vi "Fwd Kenimatics - array.vi"(4 "To":i32=7, 7 "From":i32=-1, 8 "Side":T1=enum."right", 11 "Joints":dbl[](array[numeric])=[0.0, 0.0, 0.0, 0.0, 0.0, -0.0, 0.0]) -> (0 "Matrix":T2 format="%.3f", 3 "Position":dbl[](array[numeric]) format="%.3f")   [LabVIEW 2013]
uses:
  <vilib>/Analysis/Matrix/Datatypes/RealMatrix.ctl
  ROS/Code/SubVIs/BaxterSide.ctl
  <vilib>/Analysis/Matrix/Numeric/Conversions/Array To Matrix - RA2.vi
  <vilib>/Analysis/Matrix/Numeric/Conversions/Matrix To Array - RM.vi
  <vilib>/Analysis/Matrix/Numeric/Multiply/Multiply - RM,RM.vi
  <vilib>/Analysis/Matrix/NI_Matrix.lvlib
panel:
  out "Individual":dbl[][][](array[numeric])=[[[1.0, 0.0, 0.0, 69.0], [0.0, 6.123233995736766e-17, 1.0, 0.0], [0.0, -1.0, 6.123233995736766e-17, 270.35], [0.0, 0.0, 0.0, 1.0]], [[6.123233995736766e-17, -6.123233995736766e-17, 1.0, 0.0], [1.0, 3.749399456654644e-33, -6.123233995736766e-17, 0.0], [0.0, 1.0, 6.123233995736766e-17, 0.0], [0.0, 0.0, 0.0, 1.0]], [[1.0, 0.0, 0.0, 69.0], [0.0, 6.123233995736766e-17, 1.0, 0.0], [0.0, -1.0, 6.123233995736766e-17, 364.35], [0.0, 0.0, 0.0, 1.0]], [[1.0, 0.0, 0.0, 0.0], [0.0, 6.123233995736766e-17, -1.0, 0.0], [0.0, 1.0, 6.123233995736766e-17, 0.0], [0.0, 0.0, 0.0, 1.0]], [[1.0, 0.0, 0.0, 10.0], [0.0, 6.123233995736766e-17, 1.0, 0.0], [0.0, -1.0, 6.123233995736766e-17, 374.29], [0.0, 0.0, 0.0, 1.0]], [[1.0, 0.0, 0.0, 0.0], [0.0, 6.123233995736766e-17, -1.0, 0.0], [0.0, 1.0, 6.123233995736766e-17, 0.0], [0.0, 0.0, 0.0, 1.0]], [[1.0, 0.0, 0.0, 0.0], [0.0, 1.0, 0.0, 0.0], [0.0, 0.0, 1.0, 229.525], [0.0, 0.0, 0.0, 1.0]]] format="%.3f"
  in  "D-H":cluster{"D":dbl, "R":dbl, "Rz":dbl, "Rx":dbl}[](array[cluster])=[{"D"=270.35, "R"=69.0, "Rz"=0.0, "Rx"=-90.0}, {"D"=0.0, "R"=0.0, "Rz"=90.0, "Rx"=90.0}, {"D"=364.35, "R"=69.0, "Rz"=0.0, "Rx"=-90.0}, {"D"=0.0, "R"=0.0, "Rz"=0.0, "Rx"=90.0}, {"D"=374.29, "R"=10.0, "Rz"=0.0, "Rx"=-90.0}, {"D"=0.0, "R"=0.0, "Rz"=0.0, "Rx"=90.0}, {"D"=229.525, "R"=0.0, "Rz"=0.0, "Rx"=0.0}]
  # "Does not include gripper\nFrom Base to Tool Plate"
  # "0->1\n\n1->2\n\n2->3\n\n3->4\n\n4->5\n\n5->6\n\n6->gripper"
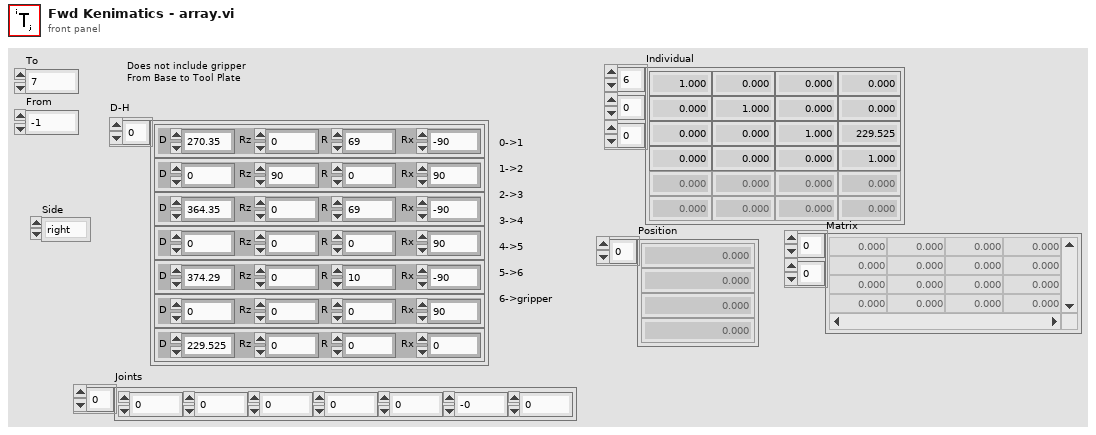
[diagram p1: front panel]
types:
  T1 = typedef "BaxterSide.ctl" = enum16{"left", "right"}
  T2 = typedef "NI_Matrix.lvlib/RealMatrix.ctl" = dbl[][]
  T3 = cluster{"Real Matrix":T2, "Real Matrix":T2, "A * B":dbl[][][]}
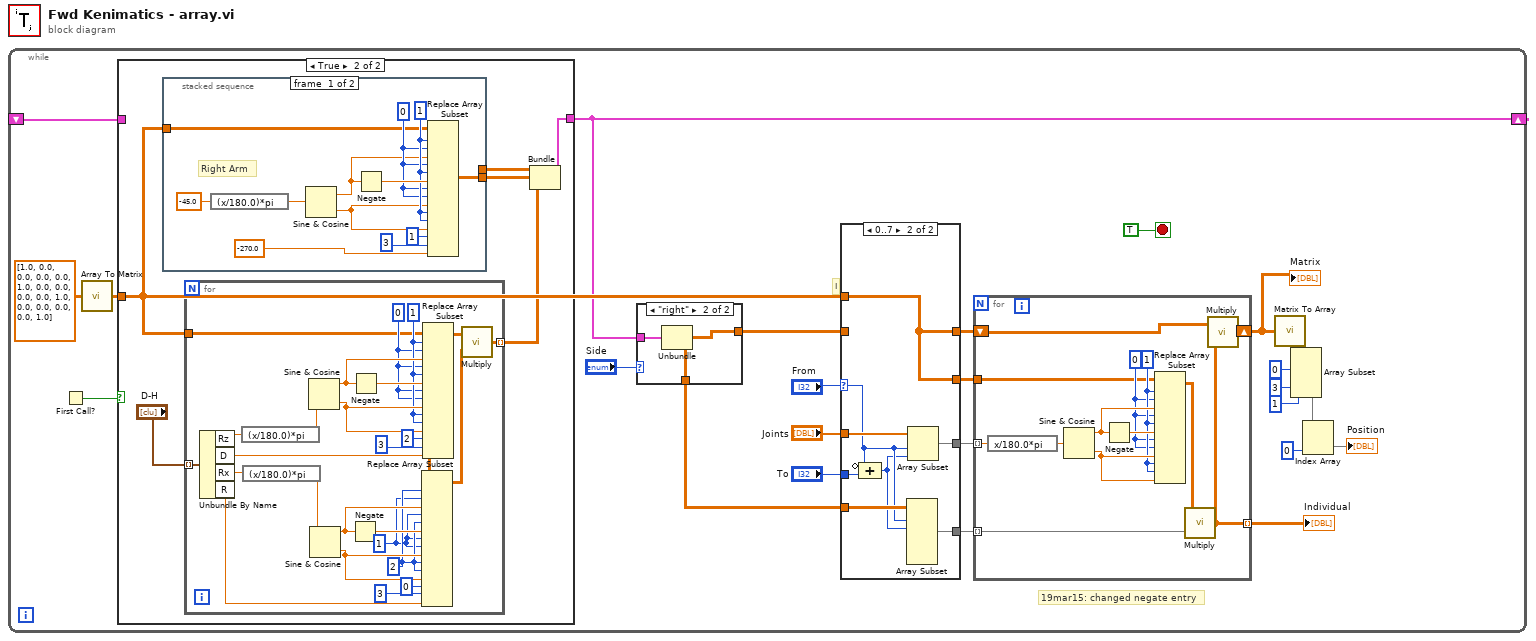
[diagram p0: block diagram]
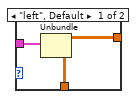
[diagram p2: hidden frame]
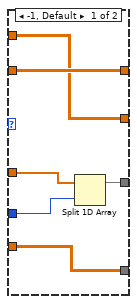
[diagram p3: hidden frame]
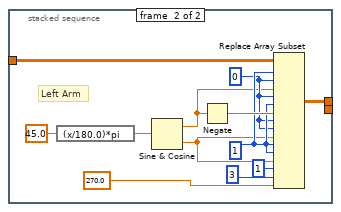
[diagram p5: hidden frame]
diagram:
  n1 = while {
    shift-right: [w4] -> _
    shift-left: _ -> [w15]
    stop <- TRUE stop-if-true
    w21 = 3 ("length")
    # "19mar15: changed negate entry"
    # "I"
    n2 = First Call?() -> (First Call?: T/F=w16:bool)
    n3 = call-poly <vilib>:"Array To Matrix.vi"("Real 2D Array"=dbl[][] [[1.0, 0.0, 0.0, 0.0], [0.0, 1.0, 0.0, 0.0], [0.0, 0.0, 1.0, 0.0], [0.0, 0.0, 0.0, 1.0]]) -> ("Real Matrix"=w7:T2)
    n4 = case shown="True" w16 {
      tunnel: [w46 w52] -> w4
      tunnel: w15 -> [w46 _]
      tunnel: w7 -> [_ w49]
      frame False {
      }
      frame True {
        n5 = stacked-sequence {
          tunnel: [w54 _] -> w51
          tunnel: w49 -> [w53 w66]
          tunnel: [_ w65] -> w47
          frame #0 {
            w61 = 1 ("index (row)")
            w60 = 0 ("disabled index (row)")
            # "Right Arm"
            n6 = expression code="(x/180.0)*pi" ("degrees to radians")(-45.0 ("Rz")) -> (w64:dbl)
            n7 = Sine & Cosine(0:w64) -> (1:w57:dbl, 2:w56:dbl)
            n8 = Negate(x=w57) -> (-x=w62:dbl)
            n9 = Replace Array Subset(array=w53, new element #1=w57, index (row) #1=w61, index (col) #1=w60, new element #2=w62, index (row) #2=w60, index (col) #2=w61, new element #3=w56, index (row) #3=w60, index (col) #3=w60, new element #4=w56, index (row) #4=w61, index (col) #4=w61, new element #5=-270.0 ("new element/submatrix"), index (row) #5=1 ("index (row)"), index (col) #5=3 ("disabled index (col)")) -> (w54:T2)
          }
          frame #1 {
            w73 = 1 ("index (row)")
            w72 = 0 ("disabled index (row)")
            # "Left Arm"
            n10 = expression code="(x/180.0)*pi" ("degrees to radians")(45.0 ("Rz")) -> (w76:dbl)
            n11 = Sine & Cosine(0:w76) -> (1:w69:dbl, 2:w68:dbl)
            n12 = Negate(x=w69) -> (-x=w74:dbl)
            n13 = Replace Array Subset(array=w66, new element #1=w69, index (row) #1=w73, index (col) #1=w72, new element #2=w74, index (row) #2=w72, index (col) #2=w73, new element #3=w68, index (row) #3=w72, index (col) #3=w72, new element #4=w68, index (row) #4=w73, index (col) #4=w73, new element #5=270.0 ("new element/submatrix"), index (row) #5=1 ("index (row)"), index (col) #5=3 ("disabled index (col)")) -> (w65:T2)
          }
        }
        n14 = for {
          tunnel: "D-H" -> [w78] mode=indexing
          tunnel: [w82] -> w50 mode=indexing
          tunnel: w49 -> [w83]
          w93 = 2 ("index (row)")
          w92 = 1 ("disabled index (row)")
          w98 = 1 ("index (row)")
          w97 = 0 ("disabled index (row)")
          n15 = Unbundle By Name(w78) -> ("Rz"=w77:dbl, "D"=w91:dbl, "Rx"=w80:dbl, "R"=w87:dbl)
          n16 = expression code="(x/180.0)*pi" ("degrees to radians")(w77) -> (w81:dbl)
          n17 = expression code="(x/180.0)*pi" ("degrees to radians")(w80) -> (w79:dbl)
          n18 = Sine & Cosine(0:w81) -> (1:w99:dbl, 2:w101:dbl)
          n19 = Sine & Cosine(0:w79) -> (1:w94:dbl, 2:w96:dbl)
          n20 = Negate(x=w94) -> (-x=w95:dbl)
          n21 = Negate(x=w99) -> (-x=w100:dbl)
          n22 = Replace Array Subset(array=w83, new element #1=w94, index (row) #1=w93, index (col) #1=w92, new element #2=w95, index (row) #2=w92, index (col) #2=w93, new element #3=w96, index (row) #3=w92, index (col) #3=w92, new element #4=w96, index (row) #4=w93, index (col) #4=w93, new element #5=w87, index (row) #5=0 ("disabled index (row)"), index (col) #5=3 ("disabled index (col)")) -> (w84:T2)
          n23 = Replace Array Subset(array=w83, new element #1=w99, index (row) #1=w98, index (col) #1=w97, new element #2=w100, index (row) #2=w97, index (col) #2=w98, new element #3=w101, index (row) #3=w97, index (col) #3=w97, new element #4=w101, index (row) #4=w98, index (col) #4=w98, new element #5=w91, index (row) #5=2 ("index (row)"), index (col) #5=3 ("disabled index (col)")) -> (w85:T2)
          n24 = call-poly <vilib>:"Multiply.vi"("Real Matrix B"=w84, "Real Matrix A"=w85) -> ("A * B"=w82:T2)
        }
        n25 = Bundle("Real Matrix"=w47, "Real Matrix"=w51, "A * B"=w50) -> (w52:T3)  [unwired: 1 in]
      }
    }
    n26 = case shown="\"right\"" "Side" {
      tunnel: w4 -> [w28 w31]
      tunnel: [w26 w30] -> w3
      tunnel: [w27 w29] -> w2
      frame "left", Default {
        n27 = Unbundle(w28) -> ("Real Matrix"=w26:T2, "A * B"=w27:dbl[][][])  [unwired: 1 out]
      }
      frame "right" {
        n28 = Unbundle(w31) -> ("Real Matrix"=w30:T2, "A * B"=w29:dbl[][][])  [unwired: 1 out]
      }
    }
    n29 = case shown="0..7" "From" {
      selector: "From" -> [_ w41]
      tunnel: [w33 w43] -> w13
      tunnel: w3 -> [w37 _]
      tunnel: [w37 w38] -> w12
      tunnel: "Joints" -> [w35 w44]
      tunnel: "To" -> [w34 w45]
      tunnel: w2 -> [w36 w42]
      tunnel: [w36 w39] -> w9
      tunnel: w7 -> [w32 w38]
      tunnel: [w32 w38] -> w6
      frame -1, Default {
        n30 = Split 1D Array(array=w35, index=w34) -> (first subarray=w33:dbl[])  [unwired: 1 out]
      }
      frame 0..7 {
        n31 = Compound Arithmetic op=ADD(invert w41, w45) -> (w40:i32)
        n32 = Array Subset(array=w42, index (dim 0)=w41, length (dim 0)=w40) -> (w39:dbl[][][])  [unwired: 4 in]
        n33 = Array Subset(array=w44, index=w41, length=w40) -> (w43:dbl[])
      }
    }
    n34 = for {
      tunnel: w13 -> [w103] mode=indexing
      tunnel: [w105] -> w25 mode=indexing
      shift-right: [w109] -> w1
      shift-left: w12 -> [w106]
      tunnel: w6 -> [w107]
      tunnel: w9 -> [w102] mode=indexing
      w111 = 1 ("index (row)")
      w110 = 0 ("disabled index (row)")
      n35 = expression code="x/180.0*pi" ("degrees to radians")(w103) -> (w104:dbl)
      n36 = Sine & Cosine(0:w104) -> (1:w112:dbl, 2:w114:dbl)
      n37 = Negate(x=w112) -> (-x=w113:dbl)
      n38 = Replace Array Subset(array=w107, new element #1=w112, index (row) #1=w111, index (col) #1=w110, new element #2=w113, index (row) #2=w110, index (col) #2=w111, new element #3=w114, index (row) #3=w110, index (col) #3=w110, new element #4=w114, index (row) #4=w111, index (col) #4=w111) -> (w108:T2)
      n39 = call-poly <vilib>:"Multiply.vi"("Real Matrix B"=w102, "Real Matrix A"=w108) -> ("A * B"=w105:T2)
      n40 = call-poly <vilib>:"Multiply.vi"("Real Matrix B"=w105, "Real Matrix A"=w106) -> ("A * B"=w109:T2)
    }
    "Individual" <- w25
    "Matrix" <- w1
    n41 = call-poly <vilib>:"Matrix To Array.vi"("Real Matrix"=w1) -> ("Real 2D Array"=w24:dbl[][])
    n42 = Array Subset(array=w24, index (row)=0 ("index"), length (row)=w21, index (col)=w21, length (col)=1 ("length")) -> (w20:dbl[][])
    n43 = Index Array(array=w20, index (col)=0 ("disabled index (col)")) -> (element=→"Position":dbl[])  [unwired: 1 in]
  }
